vi "ErrorsGlobal.vi"() -> ()   [LabVIEW 2010]
panel:
  out "Errors report":string
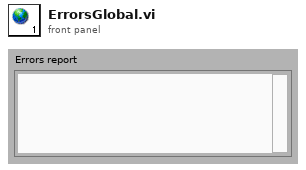
[diagram p1: front panel]
diagram:
